vi "TEST - Split Cluster TD.vi"(8 "error in (no error)":errorcluster) -> (0 "error out":errorcluster, 2 "pass":bool)   [LabVIEW 2020]
uses:
  source/library/oglib_lvdata.lvlib
  source/library/Type Descriptor.ctl
panel:
  out "Failures":T2(array[cluster])
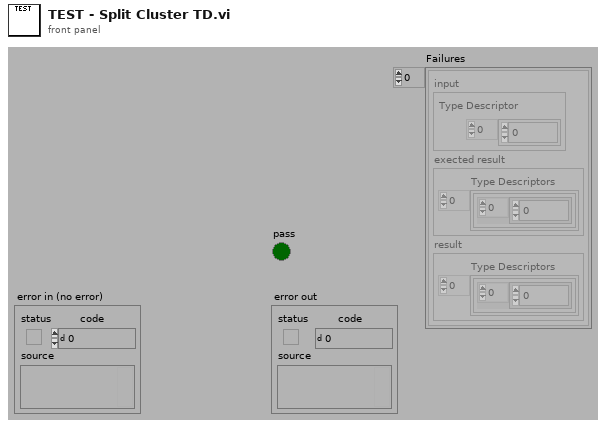
[diagram p1: front panel]
types:
  T1 = typedef "oglib_lvdata.lvlib/Type Descriptor.ctl" = i16[]
  T2 = cluster{"input":cluster{"Type Descriptor":T1}, "exected result":cluster{"Type Descriptors":cluster{"Type Descriptor":T1}[]}, "result":cluster{"Type Descriptors":cluster{"Type Descriptor":T1}[]}}[]
  T3 = cluster{"input":cluster{"Type Descriptor":T1}, "exected result":cluster{"Type Descriptors":cluster{"Type Descriptor":T1}[]}, "result":cluster{"Type Descriptors":cluster{"Type Descriptor":T1}[]}}
  T4 = typedef "Type Descriptor.ctl" = i16[]
  T5 = cluster{"Type Descriptors":cluster{"Type Descriptor":T1}[]}
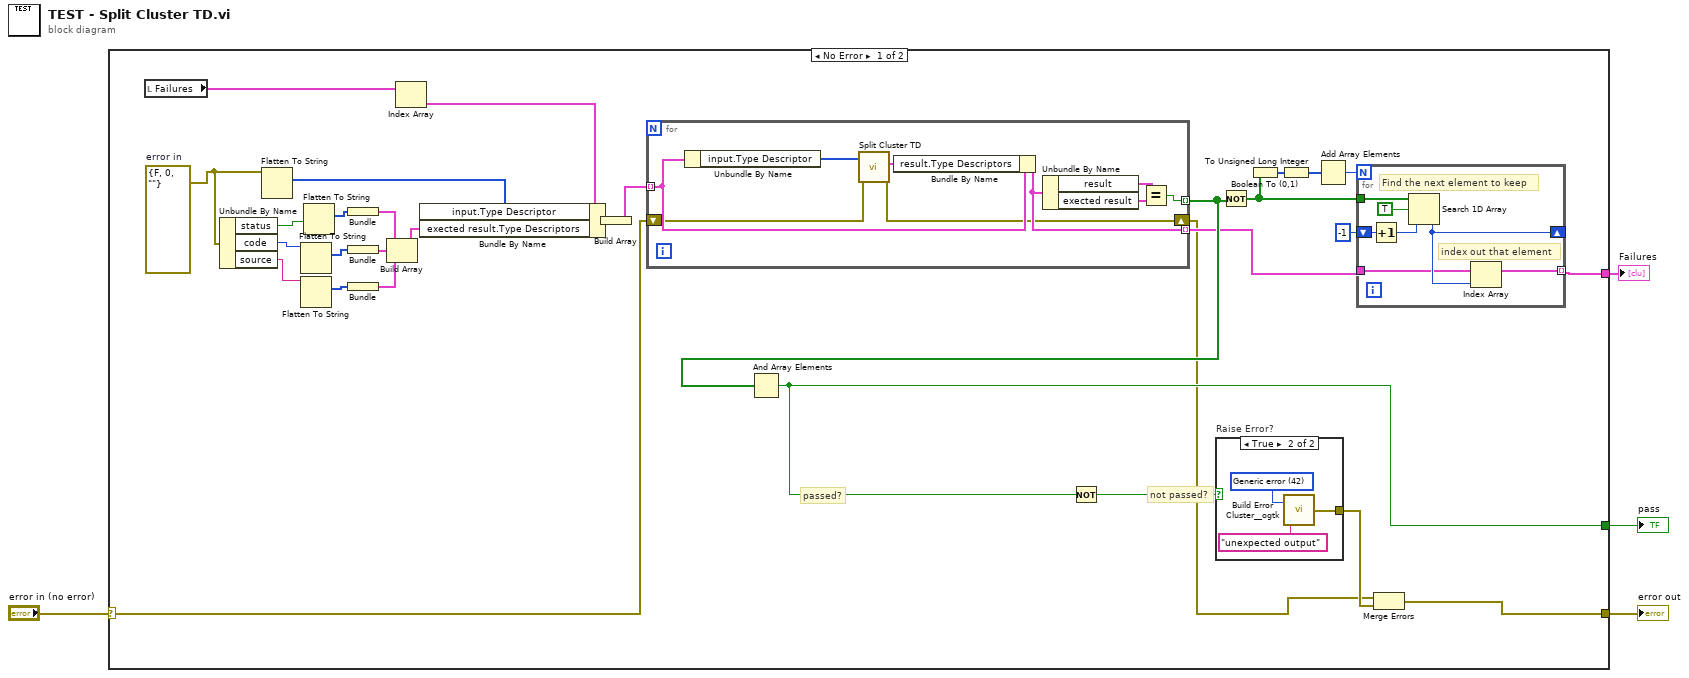
[diagram p0: block diagram]
diagram:
  n1 = case shown="No Error" "error in (no error)" {
    selector: "error in (no error)" -> [w20 w54]
    tunnel: [w31 _] -> w4
    tunnel: [w34 w54] -> w2
    tunnel: [w23 _] -> w1
    frame No Error {
      w15 = errorcluster {"status"=FALSE, "code"=0, "source"=""}  # error in
      # "not passed?"
      # "passed?"
      n2 = local read "Failures"() -> (w18:T2)
      n3 = Unbundle By Name(w15) -> ("status"=w14:bool, "code"=w6:i32, "source"=w5:string)
      n4 = Flatten To String(anything=w15) -> (type string=w16:i16[])  [unwired: 3 in, 2 out]
      n5 = Flatten To String(anything=w6) -> (type string=w12:i16[])  [unwired: 3 in, 2 out]
      n6 = Flatten To String(anything=w5) -> (type string=w11:i16[])  [unwired: 3 in, 2 out]
      n7 = Flatten To String(anything=w14) -> (type string=w13:i16[])  [unwired: 3 in, 2 out]
      n8 = Bundle("type string"=w13) -> (w10:cluster{"type string":i16[]})  [unwired: 1 in]
      n9 = Bundle("type string"=w12) -> (w9:cluster{"type string":i16[]})  [unwired: 1 in]
      n10 = Bundle("type string"=w11) -> (w8:cluster{"type string":i16[]})  [unwired: 1 in]
      n11 = Build Array(w10, w9, w8) -> (w7:cluster{"type string":i16[]}[])
      n12 = Index Array(array=w18) -> (element=w17:T3)  [unwired: 1 in]
      n13 = Bundle By Name(cluster=w17, "input.Type Descriptor"=w16, "exected result.Type Descriptors"=w7) -> (w22:T3)
      n14 = Build Array(w22) -> (w21:T2)
      n15 = for {
        tunnel: w21 -> [w49] mode=indexing
        tunnel: [w50] -> w25 mode=indexing
        tunnel: [w48] -> w24 mode=indexing
        shift-right: [w44] -> w19
        shift-left: w20 -> [w45]
        n16 = Unbundle By Name(w49) -> ("input.Type Descriptor"=w43:T1)
        n17 = call "Split Cluster TD.vi"("error in (no error)"=w45, "Type Descriptor"=w43) -> ("error out"=w44:errorcluster, "Type Descriptors"=w42:cluster{"Type Descriptor":T4}[])  [unwired: 8 in]
        n18 = Bundle By Name(cluster=w49, "result.Type Descriptors"=w42) -> (w48:T3)
        n19 = Unbundle By Name(w48) -> ("result"=w47:T5, "exected result"=w46:T5)
        n20 = Equal?(x=w47, y=w46) -> (x = y?=w50:bool)
      }
      n21 = And Array Elements(Boolean array=w25) -> (logical AND=w31:bool)
      n22 = Not(x=w31) -> (.not. x?=w32:bool)
      n23 = case "Raise Error?" shown="True" w32 {
        tunnel: [_ w51] -> w33
        frame False {
        }
        frame True {
          w52 = 42 items=["No error", "Argument error", "Memory is full", "Out of zone", "End of file", "File already open", "Generic file I/O error", "File not found", "File permission error", "Disk is full", "Duplicate path", "Too many files open", "System feature not enabled", "Resource file not found", "Cannot add resource", "Resource not found", "Image not found", "Image memory error", "Pen does not exist", "Config type invalid", "Config token not found", "Config parse error", "Config memory error", "Bad external code format", "Bad external code offset", "External code not present", "Null window", "Destroy window error", "Null menu", "Print aborted", "Bad print record", "Print driver error", "Windows error during printing", "Memory error during printing", "Print dialog error", "Generic print error", "Invalid device refnum", "Device not found", "Device parameter error", "Device unit error", "Cannot open device", "Device call aborted", "Generic error", "Cancelled by user", "Object ID too low", "Object ID too high", "Object not in heap", "Unknown heap", "Unknown object (invalid DefProc)", "Unknown object (DefProc not in table)", "Message out of range", "Invalid (null) method", "Unknown message", "Manager call not supported", "Bad address", "Network operation in progress", "Network operation timed out", "Connection is busy", "Network attribute not supported", "Network error", "Address in use", "System out of memory", "Connection aborted", "Connection refused", "Not connected", "Already connected", "Connection closed", "Initialization error (interapplication manager)", "Bad occurrence", "Wait on unbound occurrence handler", "Occurrence queue overflow", "Datalog type conflict", "Unused", "Unrecognized type (interapplication manager)", "Memory corrupt", "Failed to make temporary DLL", "Old CIN version", "Drag socket not found", "Failed to load drop-object", "Failed to register OLE object", "Failed to release OLE object", "Format specifier type mismatch", "Unknown format specifier", "Too few format specifiers", "Too many format specifiers", "Scan failed", "Newer CIN version", "Error converting to variant", "Runtime menu error", "Password tampered", "Variant attribute not found", "Incompatible variant data type", "Event data is not available", "Event Store is not present", "Occurrence is not found", "Event Queue is not created", "Event info is not available", "Refnum passed is NULL", "Error retrieving Class GUID", "Error retrieving CoClass GUID", "Error retrieving TypeLib GUID.", "Bad built application magic bytes.", "Specific driver is different from the specific driver associated with the Logical Name.", "There is no session opened to the class driver.", "Max Error", "MAX - Error with config objects", "MAX - Error loading configuration", "MAX - Group not supported"]
          n24 = call <userlib>:"Build Error Cluster__ogtk.vi"("String to Prepend to source (\"\")"="unexpected output" ("String to Prepend to source (\"\")"), "code"=w52) -> ("error out"=w51:errorcluster)
        }
      }
      n25 = Not(x=w25) -> (.not. x?=w27:bool[])
      n26 = Boolean To (0,1)(Boolean=w27) -> (0, 1=w28:i16[])
      n27 = To Unsigned Long Integer(number=w28) -> (unsigned 32bit integer=w26:u32[])
      n28 = Add Array Elements(numeric array=w26) -> (sum=w29:u32)
      n29 = for {
        N: w29 -> [_]
        tunnel: w24 -> [w37]
        tunnel: w27 -> [w41]
        shift-right: [w38] -> _
        shift-left: -1 ("start index (0)") -> [w39]
        tunnel: [w36] -> w23 mode=indexing
        # "index out that element"
        # "Find the next element to keep"
        n30 = Increment(x=w39) -> (x+1=w35:i32)
        n31 = Search 1D Array(1D array=w41, element=TRUE, start index (0)=w35) -> (index of element=w38:i32)
        n32 = Index Array(array=w37, index=w38) -> (element=w36:T3)
      }
      n33 = Merge Errors(w19, w33) -> (w34:errorcluster)
    }
    frame Error {
    }
  }
  "pass" <- w4
  "error out" <- w2
  "Failures" <- w1
